vi "CoriolisMain.vi"() -> ()   [LabVIEW 2021]
panel:
  out "Array 2":i32[][](array[numeric])
  out "Array":dbl[][](array[numeric])
  out "time stamp":timestamp
  out "current time":timestamp
  out "appended path":path
  out "string":string
  in  "python version":string="3.6"
  out "error out":errorcluster
  in  "error in (no error)":errorcluster
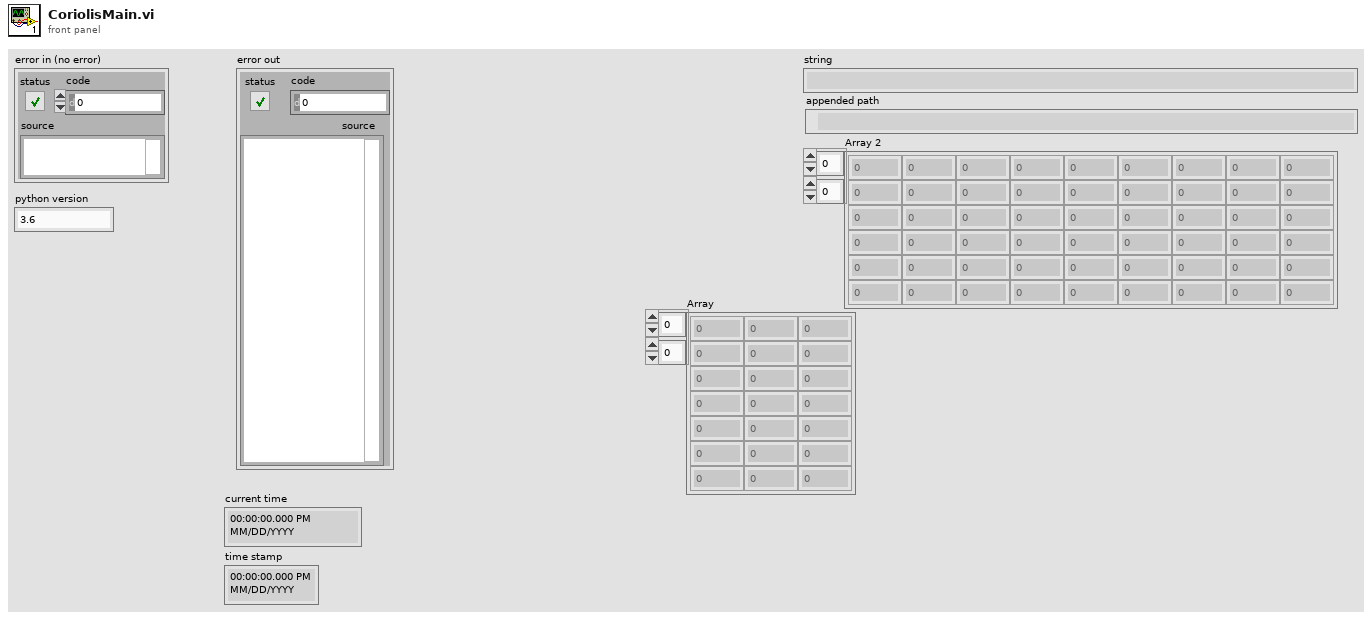
[diagram p1: front panel]
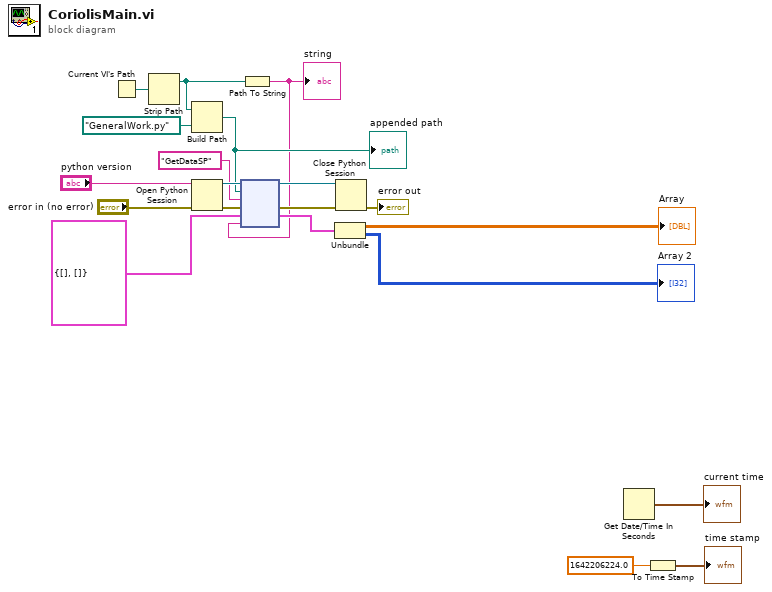
[diagram p0: block diagram]
diagram:
  n1 = Current VI's Path() -> (path=w11:path)
  n2 = Strip Path(path=w11) -> (stripped path=w9:path)  [unwired: 1 out]
  n3 = Build Path(base path=w9, name or relative path=path "GeneralWork.py" ("python path")) -> (appended path=w13:path)
  "appended path" <- w13
  n4 = Open Python Session(python version="python version", 3:"error in (no error)") -> (session out=w18:refnum<k35>, error out=w17:errorcluster)  [unwired: 1 in]
  n5 = Path To String(path=w9) -> (string=w1:string)
  "string" <- w1
  n6 = node(w18, w13, "GetDataSP" ("function name in"), w17, cluster{dbl[][], i32[][]} {[], []}, w1) -> (w20:refnum<k35>, w19:errorcluster, w3:cluster{dbl[][], i32[][]})  [unwired: 1 in, 2 out]
  n7 = Unbundle(w3) -> (→"Array":dbl[][], →"Array 2":i32[][])
  n8 = Close Python Session(session in=w20, error in=w19) -> (11:→"error out":errorcluster)
  n9 = Get Date/Time In Seconds() -> (seconds since 1Jan1904=→"current time":timestamp)
  n10 = To Time Stamp(1:1642206224.0 ("number")) -> (0:→"time stamp":timestamp)
